vi "N6701A_SetVoltageCurrent.vi"(6 "Current Limit (amps)":dbl format="%^.3e", 7 "Voltage Level":dbl format="%^.3e", 8 "error in (no error)":errorcluster, 9 "Behavior (0: Regulatory Limit)":i32(ring) items=["Regulatory Limit", "Trip Limit"], 10 "Channel Name (1)":string="1", 11 "VISA resource name":refnum<visa-resource-name>) -> (0 "error out":errorcluster)   [LabVIEW 2015]
doc: "This VI will set the Voltage taking into acount the polarity and the Current of the Power Supply\n\nThe input is an array of setting to allow the user to set all or one channel on as many devices as required"
uses:
  <instrlib>/Agilent N6700 Series/Agilent N6700 Series.lvlib
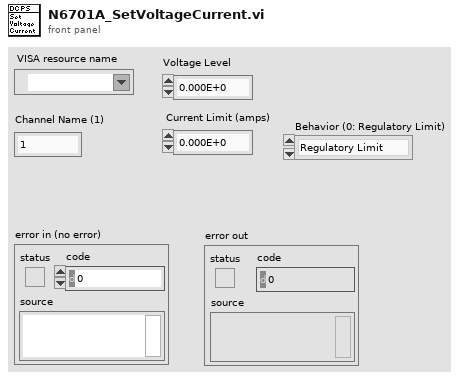
[diagram p1: front panel]
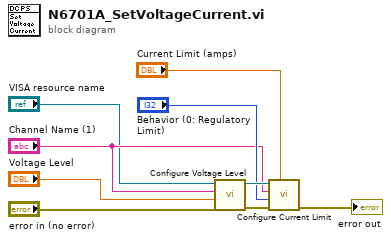
[diagram p0: block diagram]
diagram:
  n1 = call <instrlib>:"Configure Voltage Level.vi"("error in (no error)"="error in (no error)", "Level  (0.0 volts)"="Voltage Level", "Channel Name (1)"="Channel Name (1)", "VISA resource name"="VISA resource name") -> ("error out"=w8:errorcluster, "VISA resource name out"=w9:refnum<visa-resource-name>)  [unwired: 6 in]
  n2 = call <instrlib>:"Configure Current Limit.vi"("Limit (0.0 amps)"="Current Limit (amps)", "error in (no error)"=w8, "Behavior (0: Regulatory Limit)"="Behavior (0: Regulatory Limit)", "Channel Name (1)"="Channel Name (1)", "VISA resource name"=w9) -> ("error out"=→"error out":errorcluster)  [unwired: 5 in, 1 out]
